vi "SumTimeSpendAnalyze_171213.vi"(11 "Clean data array":dbl[][](array[numeric])) -> (3 "Item Names":string[][](array[string]))   [LabVIEW 2016]
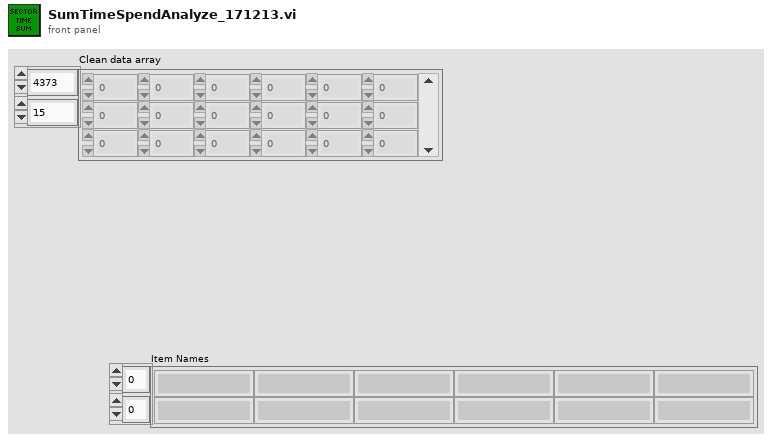
[diagram p1: front panel]
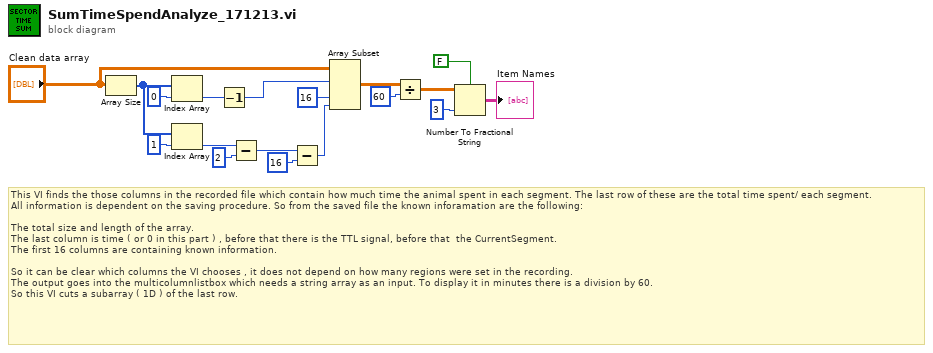
[diagram p0: block diagram]
diagram:
  # "This VI finds the those columns in the recorded file which contain how much time the animal spent in each segment. The last row of these are the total time spent/ each segment.\nAll information is dependent on the saving procedure. So from the saved file the known inforamation are the following:\n\nThe total size and length of the array.\nThe last column is time ( or 0 in this part ) , before that there is the TTL signal, before that  the CurrentSegment.\nThe first 16 columns are containing known information.\n\nSo it can be clear which columns the VI chooses , it does not depend on how many regions were set in the recording.\nThe output goes into the multicolumnlistbox which needs a string array as an input. To display it in minutes there is a division by 60. \nSo this VI cuts a subarray ( 1D ) of the last row."
  n1 = Array Size(array="Clean data array") -> (size(s)=w15:i32[])
  n2 = Index Array(array=w15, index=0) -> (element=w16:i32)
  n3 = Index Array(array=w15, index=1) -> (element=w13:i32)
  n4 = Decrement(x=w16) -> (x-1=w7:i32)
  n5 = Subtract(x=w13, y=2) -> (x-y=w11:i32)
  n6 = Subtract(x=w11, y=16 ("index")) -> (x-y=w9:i32)
  n7 = Array Subset(array="Clean data array", index (row)=w7, index (col)=16 ("index"), length (col)=w9) -> (w3:dbl[][])  [unwired: 1 in]
  n8 = Divide(x=w3, y=60 ("index")) -> (x/y=w4:dbl[][])
  n9 = Number To Fractional String(use system decimal point (T)=FALSE, number=w4, precision (6)=i16 3) -> (F-format string=→"Item Names":string[][])  [unwired: 1 in]
